vi "利用极坐标求直角三角形斜边.vi"(1 "b":dbl=4.0, 2 "a":dbl=3.0) -> (0 "c":dbl=5.0)   [LabVIEW 2012, in "几何工具.lvlib"]
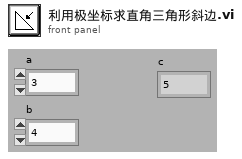
[diagram p1: front panel]
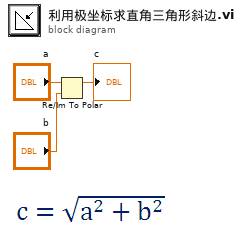
[diagram p0: block diagram]
diagram:
  n1 = Re/Im To Polar(2:"b", 3:"a") -> (1:→"c":dbl)  [unwired: 1 out]
